vi "Yokogawa GX20 Acquire Continuous Measurement Data Example Ether_RS232C Single.vi"() -> ()   [LabVIEW 2020]
doc: "This example shows how to configure multiple channels and acquire measurement data from multiple channels."
uses:
  <instrlib>/Yokogawa GX Series/Public/Data/Read Measurement Data (Analog NChan).vi
  <instrlib>/Yokogawa GX Series/Yokogawa GX Series.lvlib
panel:
  in  "Serial Configuration":T1={"Baud Rate"=9600, "Parity"=2, "Data Bits"=8, "Flow Control"=0} {"Flow Control" items=["None", "XON/XOFF", "RTS/CTS", "XON/XOFF & RTS/CTS"]; "Data Bits" items=["7"=7, "8"=8]; "Parity" items=["None", "Odd", "Even"]; "Baud Rate" items=["1200"=1200, "2400"=2400, "4800"=4800, "9600"=9600, "19200"=19200, "38400"=38400, "57600"=57600, "115200"=115200]}
  in  "User ID (\"\")":string
  out "Ch":string[](array[string])
  out "Unit":string[](array[string])
  out "Data":dbl[](array[numeric]) format="%#_5f"
  in  "Password (\"\")":string
  in  "User Name (\"\")":string
  in  "Interval (1000)":u32=1000 min=25
  out "Date Time":timestamp=timestamp(3345116400 s since 1904-01-01) format="%<%H:%M:%S%3u\n%x>T"
  in  "End Channel (0010)":string="0010"
  in  "Start Channel (0001)":string="0001"
  in  "VISA resource name":refnum<visa-resource-name>
  in  "Stop":bool
  out "Chart":dbl[][](graph)
  # "(c) 2013-2018 Yokogawa Electric Corporation.  ALL RIGHTS RESERVED."
  # "GX/GP/GM PAPERLESS RECORDER"
  # "ms"
  # "To execute this example, do below.\n1) Attach AI module to GX/GP/GM.\n2) Do Reconfiguring the GX/GP/GM (See User's Manual 1.24.2)\n3) Run this VI with valid VISA resource name (ex: \"TCPIP::192.168.0.2::34434::SOCKET\")"
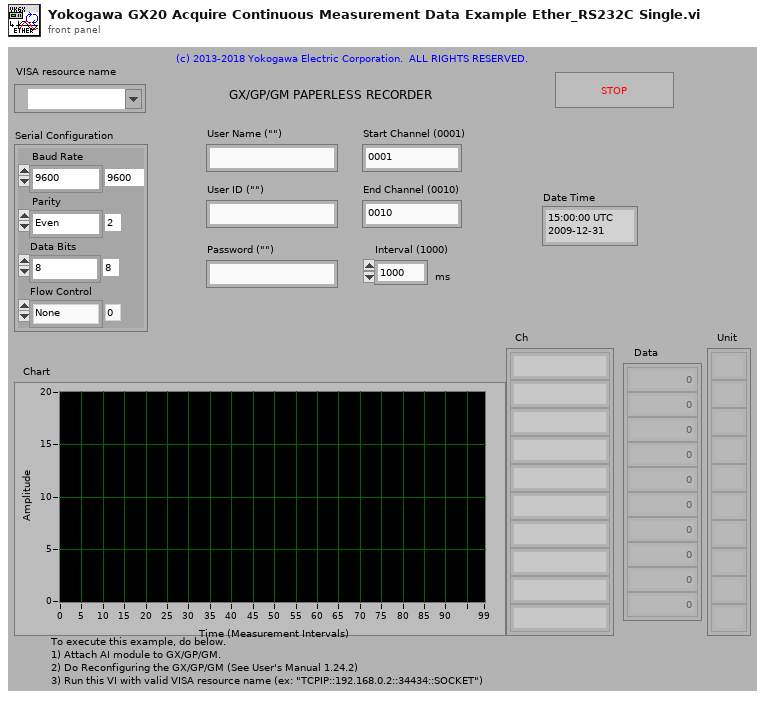
[diagram p1: front panel]
types:
  T1 = cluster{"Baud Rate":u32, "Parity":u16, "Data Bits":u16, "Flow Control":u16}
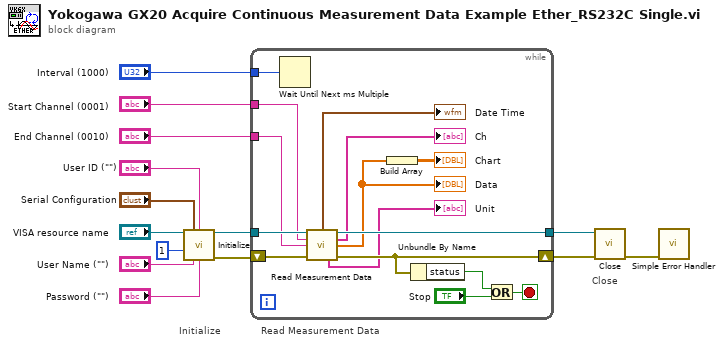
[diagram p0: block diagram]
diagram:
  # "Read Measurement Data"
  # "Close"
  # "Initialize"
  n1 = call <instrlib>:"Initialize.vi"("VISA resource name IN"="VISA resource name", "Serial Configuration"="Serial Configuration", "User ID (\"\")"="User ID (\"\")", "Serial Auth Type (0: Not Auth)"=u16 1, "User Name (\"admin\")"="User Name (\"\")", "Password (\"\")"="Password (\"\")") -> ("VISA resource name out"=w4:refnum<visa-resource-name>, "error out"=w5:errorcluster)  [unwired: 8 in]
  n2 = while {
    shift-left: w5 -> [w24]
    shift-right: [w26] -> w14
    tunnel: [w25] -> w12
    tunnel: w4 -> [w23]
    tunnel: "Interval (1000)" -> [w21]
    tunnel: "Start Channel (0001)" -> [w20]
    tunnel: "End Channel (0010)" -> [w19]
    stop <- w28 stop-if-true
    n3 = Wait Until Next ms Multiple(millisecond multiple=w21) -> ()  [unwired: 1 out]
    n4 = call-poly <instrlib>:"Read Measurement Data.vi"("VISA resource name"=w23, "Start Channel (1)"=w20, "End Channel (1)"=w19, "error in (no error)"=w24) -> ("Date Time"=→"Date Time":timestamp, "VISA resource name out"=w25:refnum<visa-resource-name>, "Channel"=→"Ch":string[], "Data"=w18:dbl[], "Unit"=→"Unit":string[], "error out"=w26:errorcluster)  [unwired: 1 in, 5 out]
    "Data" <- w18
    n5 = Build Array(w18) -> (→"Chart":dbl[][])
    n6 = Unbundle By Name(w26) -> ("status"=w27:bool)
    n7 = Or(x=w27, y="Stop") -> (x .or. y?=w28:bool)
  }
  n8 = call <instrlib>:"Close.vi"("error in (no error)"=w14, "VISA resource name"=w12) -> ("error out"=w13:errorcluster)  [unwired: 9 out]
  n9 = call <vilib>:"Simple Error Handler.vi"("error in (no error)"=w13) -> ()  [unwired: 1 in, 8 out]
